vi "RepDoc map image file type.vi"(1 "image file type (.jpg)":enum16{".jpg", ".png"}(ring)) -> (0 "image format (jpeg)":enum32{"PNG", "JPEG", "GIF"}(ring)=enum."JPEG")   [LabVIEW 2017, in "NI_ReportGenerationCore.lvlib"]
uses:
  <vilib>/Utility/NIReport.llb/NI_ReportGenerationCore.lvlib
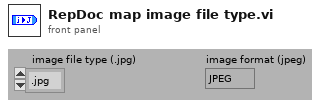
[diagram p1: front panel]
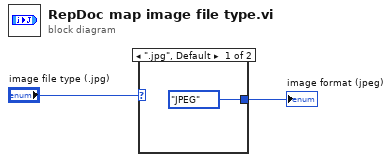
[diagram p0: block diagram]
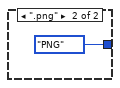
[diagram p2: hidden frame]
diagram:
  n1 = case shown="\".jpg\", Default" "image file type (.jpg)" {
    tunnel: [enum32{"PNG", "JPEG", "GIF"}."JPEG" ("Image Format (jpeg)") enum32{"PNG", "JPEG", "GIF"}."PNG" ("Image Format (jpeg)")] -> w1
    frame ".jpg", Default {
    }
    frame ".png" {
    }
  }
  "image format (jpeg)" <- w1
